vi "Initialize.vi"(8 "Error In":errorcluster, 11 "Audio Analyzer In":refnum<class "Audio Analyzer.lvclass">) -> (0 "Error Out":errorcluster, 3 "Audio Analyzer Out":refnum<class "Audio Analyzer.lvclass">)   [LabVIEW 2019, in "Audio Analyzer.lvclass"]
uses:
  Audio Analyzer.lvclass
  Process/Process.lvclass
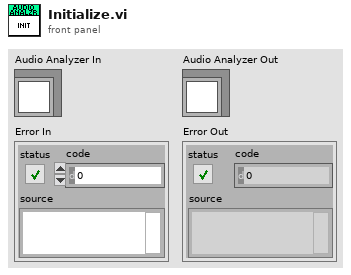
[diagram p1: front panel]
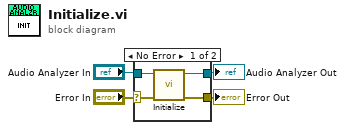
[diagram p0: block diagram]
diagram:
  n1 = case shown="No Error" "Error In" {
    selector: "Error In" -> [w8 w9]
    tunnel: [w5 w9] -> w4
    tunnel: [w6 w10] -> w3
    tunnel: "Audio Analyzer In" -> [w7 w10]
    frame No Error {
      n2 = call-parent "Initialize.vi"("Error In"=w8, "Process In"=w7) -> ("Error Out"=w5:errorcluster, "Process Out"=w6:refnum<class "Audio Analyzer.lvclass">)  [unwired: 8 in]
    }
    frame Error {
    }
  }
  "Audio Analyzer Out" <- w3
  "Error Out" <- w4
